vi "Get Program Directories.vi"() -> (0 "Program Directories":path[](array[path]))   [LabVIEW 2019, in "Control Experiment.lvclass"]
uses:
  Control Experiment.lvclass
  <vilib>/registry/registry.llb/Registry SAM.ctl
  <vilib>/registry/registry.llb/Read Registry Value Simple STR.vi
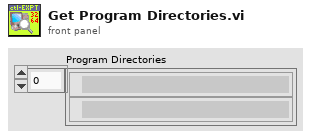
[diagram p1: front panel]
types:
  T1 = typedef "Registry SAM.ctl" = enum32{"KEY_QUERY_VALUE", "KEY_SET_VALUE", "KEY_CREATE_SUB_KEY", "KEY_ENUMERATE_SUB_KEYS", "KEY_NOTIFY", "KEY_CREATE_LINK", "KEY_READ", "KEY_WRITE", "KEY_ALL_ACCESS", "KEY_READ | KEY_WRITE"}
  T2 = typedef "Registry refnum.ctl" = refnum<k1>
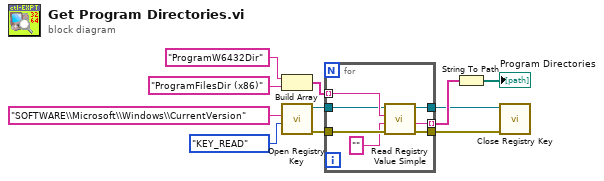
[diagram p0: block diagram]
diagram:
  n1 = Build Array("ProgramW6432Dir" ("value"), "ProgramFilesDir (x86)" ("value")) -> (w4:string[])
  n2 = call <vilib>:"Open Registry Key.vi"("security access mask (KEY_READ | KEY_WRITE)"=Registry_SAM."KEY_READ", "subkey"="SOFTWARE\\Microsoft\\Windows\\CurrentVersion") -> ("error out"=w7:errorcluster, "refnum out"=w8:T2)  [unwired: 8 in]
  n3 = for {
    tunnel: w4 -> [w14] mode=indexing
    tunnel: [w18] -> w9 mode=indexing
    tunnel: w7 -> [w17]
    tunnel: [w15] -> w5
    tunnel: w8 -> [w12]
    tunnel: [w16] -> w6
    n4 = call-poly <vilib>:"Read Registry Value Simple.vi"("error in (no error)"=w17, "default data"="", "value"=w14, "refnum"=w12) -> ("error out"=w15:errorcluster, "String/Binary data"=w18:string, "refnum out"=w16:T2)  [unwired: 2 in, 1 out]
  }
  n5 = String To Path(string=w9) -> (path=→"Program Directories":path[])
  n6 = call <vilib>:"Close Registry Key.vi"("error in (no error)"=w5, "refnum"=w6) -> ()  [unwired: 5 in, 1 out]
